vi "Get msg from mailbox.vi"(8 "error in (no error)":errorcluster, 9 "timeout ms (1000)":i32=1000, 11 "Mailbox ref in":T1) -> (0 "error out":errorcluster, 1 "Message":T2 {"Time Stamp" format="%<%H:%M:%S\n%Y/%m/%d>T"}, 2 "timed out?":bool, 3 "mailbox ref out":T1, 4 "pending messages":i32, 5 "Mailbox name":string)   [LabVIEW 2021, in "Queued messenger.lvlib"]
doc: "Receives the first message in the mailbox if there is any. If there is no message, it waits for a message till timeout. Also returns a state of mailbox."
uses:
  <userlib>/MatS libs/MatS Messenger/Queued messenger.lvlib
  <userlib>/MatS libs/MatS Messenger/TypeDefs/Mailbox ref.ctl
  <userlib>/MatS libs/MatS Messenger/TypeDefs/General message.ctl
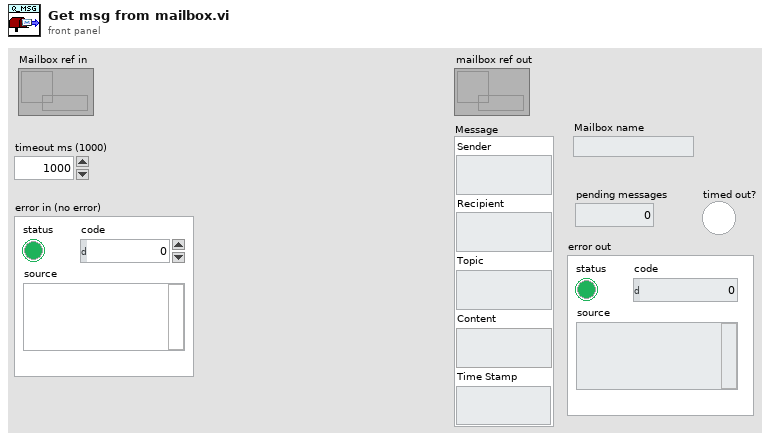
[diagram p1: front panel]
types:
  T1 = typedef "Queued messenger.lvlib/Mailbox ref.ctl" = refnum<queue>
  T2 = typedef "Queued messenger.lvlib/General message.ctl" = cluster{"Sender":string, "Recipient":string, "Topic":string, "Content":variant, "Time Stamp":timestamp}
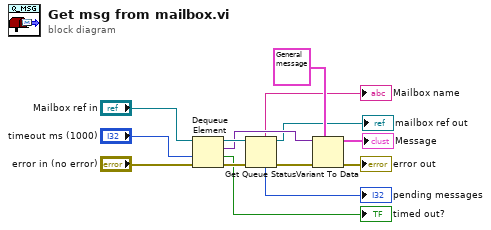
[diagram p0: block diagram]
diagram:
  n1 = Dequeue Element(queue="Mailbox ref in", timeout in ms (-1)="timeout ms (1000)", error in (no error)="error in (no error)") -> (queue out=w13:T1, element=w9:variant, timed out?=→"timed out?":bool, error out=w8:errorcluster)
  n2 = Get Queue Status(queue=w13, error in (no error)=w8) -> (queue out=→"mailbox ref out":T1, queue name=→"Mailbox name":string, error out=w7:errorcluster, # elements in queue=→"pending messages":i32)  [unwired: 1 in, 4 out]
  n3 = Variant To Data(error in=w7, type=T2 {"Sender"="", "Recipient"="", "Topic"="", "Content"=variant, "Time Stamp"=timestamp(0 s since 1904-01-01)} ("Message"), Variant=w9) -> (data=→"Message":T2, error out=→"error out":errorcluster)
